vi "spindisk_config_file.vi"(0 "config file path name":string, 1 "section":string="Excitation", 2 "common_keyname":string="ExcitationFilterPosition", 3 "error in (no error)":errorcluster, 4 "Positions":i32) -> (5 "filter list":string[](array[string]), 6 "error out":errorcluster)   [LabVIEW 2016]
uses:
  <vilib>/Utility/config.llb/Read Key (String).vi
  <vilib>/Utility/config.llb/Write Key (String).vi
  <vilib>/Utility/config.llb/NI_LVConfig.lvlib
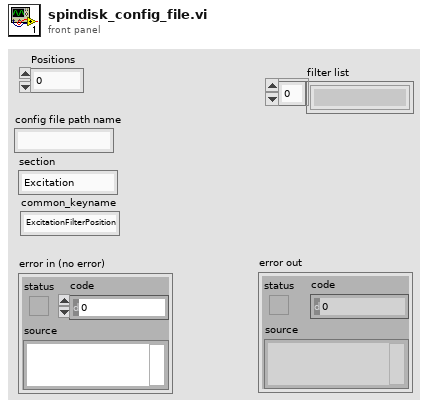
[diagram p1: front panel]
types:
  T1 = typedef "NI_LVConfig.lvlib/Config Data RefNum.ctl" = refnum<k1>
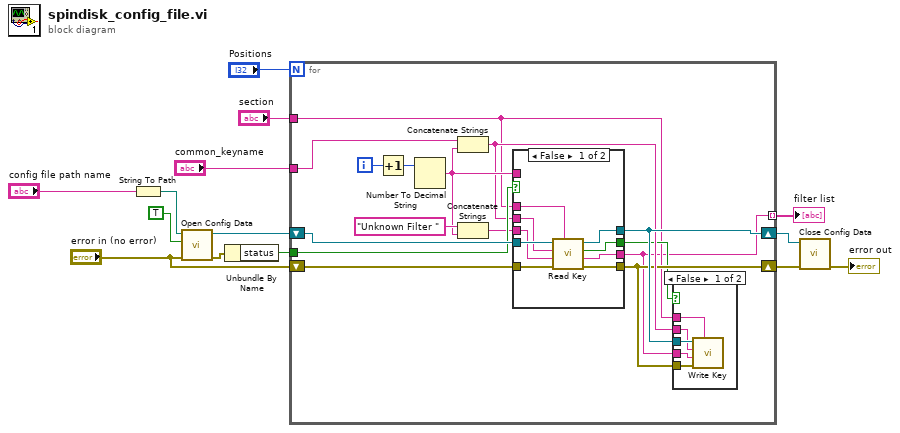
[diagram p0: block diagram]
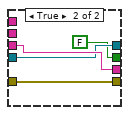
[diagram p3: hidden frame]
diagram:
  n1 = String To Path(string="config file path name") -> (path=w10:path)
  n2 = call <vilib>:"Open Config Data.vi"("error in (no error)"="error in (no error)", "create file if necessary (T)"=TRUE, "configuration file path"=w10) -> ("error out"=w12:errorcluster, "refnum"=w14:T1)  [unwired: 6 in, 1 out]
  n3 = Unbundle By Name(w12) -> ("status"=w11:bool)
  n4 = for {
    N: "Positions" -> [_]
    shift-right: [w22] -> w9
    shift-left: w14 -> [w29]
    shift-right: [w19] -> w8
    shift-left: "error in (no error)" -> [w28]
    tunnel: w11 -> [w27]
    tunnel: [w15] -> w1 mode=indexing
    tunnel: "section" -> [w17]
    tunnel: "common_keyname" -> [w16]
    i -> [w26]
    n5 = Increment(x=w26) -> (x+1=w25:i32)
    n6 = Number To Decimal String(number=w25) -> (decimal integer string=w21:string)  [unwired: 1 in]
    n7 = Concatenate Strings(w16, w21) -> (w20:string)
    n8 = Concatenate Strings("Unknown Filter " ("default value"), w21) -> (w23:string)
    n9 = case shown="False" w27 {
      tunnel: w29 -> [w43 w45]
      tunnel: [w42 w45] -> w22
      tunnel: w28 -> [w41 w47]
      tunnel: [w40 w47] -> w19
      tunnel: [w39 w46] -> w15
      tunnel: w21 -> [_ _]
      tunnel: w23 -> [w38 w46]
      tunnel: w17 -> [w37 _]
      tunnel: w20 -> [w36 _]
      tunnel: [w35 FALSE ("found?")] -> w18
      frame False {
        n10 = call-poly <vilib>:"Read Key.vi"("section"=w37, "error in (no error)"=w41, "default value"=w38, "key"=w36, "refnum"=w43) -> ("error out"=w40:errorcluster, "value"=w39:string, "found?"=w35:bool, "refnum out"=w42:T1)  [unwired: 3 in]
      }
      frame True {
      }
    }
    n11 = case shown="False" w18 {
      tunnel: w22 -> [w34 _]
      tunnel: w17 -> [w33 _]
      tunnel: w20 -> [w32 _]
      tunnel: w15 -> [w31 _]
      tunnel: w19 -> [w30 _]
      frame False {
        n12 = call-poly <vilib>:"Write Key.vi"("section"=w33, "error in (no error)"=w30, "value"=w31, "key"=w32, "refnum"=w34) -> ()  [unwired: 4 in, 3 out]
      }
      frame True {
      }
    }
  }
  "filter list" <- w1
  n13 = call <vilib>:"Close Config Data.vi"("error in (no error)"=w8, "refnum"=w9) -> ("error out"=→"error out":errorcluster)  [unwired: 8 in, 1 out]
